vi "test_data.vi"() -> ()   [LabVIEW 2014]
panel:
  out "Waveform Graph":waveform(dbl)[](graph)
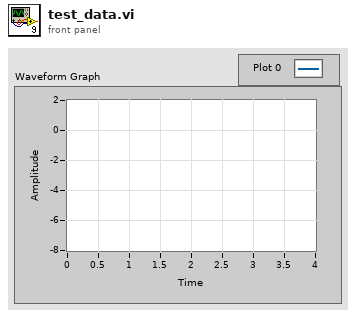
[diagram p1: front panel]
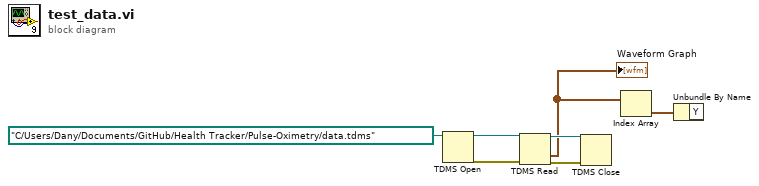
[diagram p0: block diagram]
diagram:
  n1 = TDMS Open(11:path "C:/Users/Dany/Documents/GitHub/Health Tracker/Pulse-Oximetry/data.tdms" ("file path")) -> (0:w6:errorcluster, 3:w7:refnum<k34>)  [unwired: 6 in]
  n2 = TDMS Read(0:w7, 11:w6) -> (4:w5:refnum<k34>, 10:w2:waveform(dbl)[], 15:w4:errorcluster)  [unwired: 6 in, 3 out]
  "Waveform Graph" <- w2
  n3 = TDMS Close(8:w4, 11:w5) -> ()  [unwired: 2 out]
  n4 = Index Array(array=w2) -> (element=w1:waveform(dbl))  [unwired: 1 in]
  n5 = Unbundle By Name(w1) -> ()  [unwired: 1 out]
